vi "PolarizationSimulation_Final.vi"() -> ()   [LabVIEW 2019]
uses:
  <vilib>/Analysis/NI_AALBase.lvlib
  <vilib>/Utility/xml.llb/Write to XML File(string).vi
  <vilib>/Utility/xml.llb/Read From XML File(string).vi
  Integrated ANN/Sub-VIs/Adam_data.ctl
panel:
  out "Standard \nDeviation Noise":dbl step=0.0001
  out "NN Error":dbl
  out "NN Output":dbl
  out "Saturation\nPolarization":dbl=0.8 min=0.0 max=0.99 step=0.01
  out "Signal and Fit (P) 2":cluster{dbl[], "Best Polynomial Fit":dbl[]}[](graph)
  out "NN Graph":cluster{dbl[], dbl[]}(graph)
  in  "Regularization":T1
  in  "Batch Size":i16
  out "NN Loss":dbl(graph)
  in  "Loss Function":enum16{"MSE", "MAE"}(ring)
  in  "Parameters File Path":path
  out "NN Error":dbl
  in  "Training?":bool
  out "NN Output":dbl
  in  "Speed\nMultiplier":dbl=1.0
  in  "AFP On":bool
  in  "AFP Efficiency":dbl=0.9 min=0.0 max=1.0 step=0.01
  in  "AFP Control":cluster{i32, i32}(slide)={200, 230} scale=0.0..500.0
  out "lower R-value AFP":dbl
  out "upper R-value AFP":dbl
  in  "STOP":bool
  in  "Microwave Power":dbl=1.0
  in  "Lower Fit\nParameter":dbl=-3.6
  in  "Upper Fit\nParameter":dbl=3.6
  in  "Std Dev Noise":dbl step=0.0001
  out "lower R-value":dbl
  out "upper R-value":dbl
  in  "RF Control":cluster{i32, i32}(slide)={200, 230} scale=0.0..500.0
  out "p":dbl format="%_4g"
  out "r":dbl
  in  "Saturation\nPolarization":dbl=0.8 min=0.0 max=0.99 step=0.01
  out "Reimann \nsum of Q":dbl format="%_4g"
  out "Corrected Data (Q)":cluster{dbl[], dbl[]}(graph)
  in  "Select Target Type":u16(ring)=2 items=["Test Case", "Deuteron"]
  in  "Reset":bool
  out "Total Polarization (P)":cluster{dbl, dbl}(graph)
  in  "Spin Manipulation\nPower Factor":dbl=0.005
  in  "Decay Spin\nManipulation":bool
  out "Reimann\nsum of P":dbl format="%_4g"
  out "Corrected Data (P)":cluster{dbl[], dbl[]}[](graph)
  out "Signal and Fit (P)":cluster{dbl[], "Best Polynomial Fit":dbl[]}[](graph)
  in  "Positive\nPolarization":bool
  in  "Microwave on":bool
  # "Neural Network"
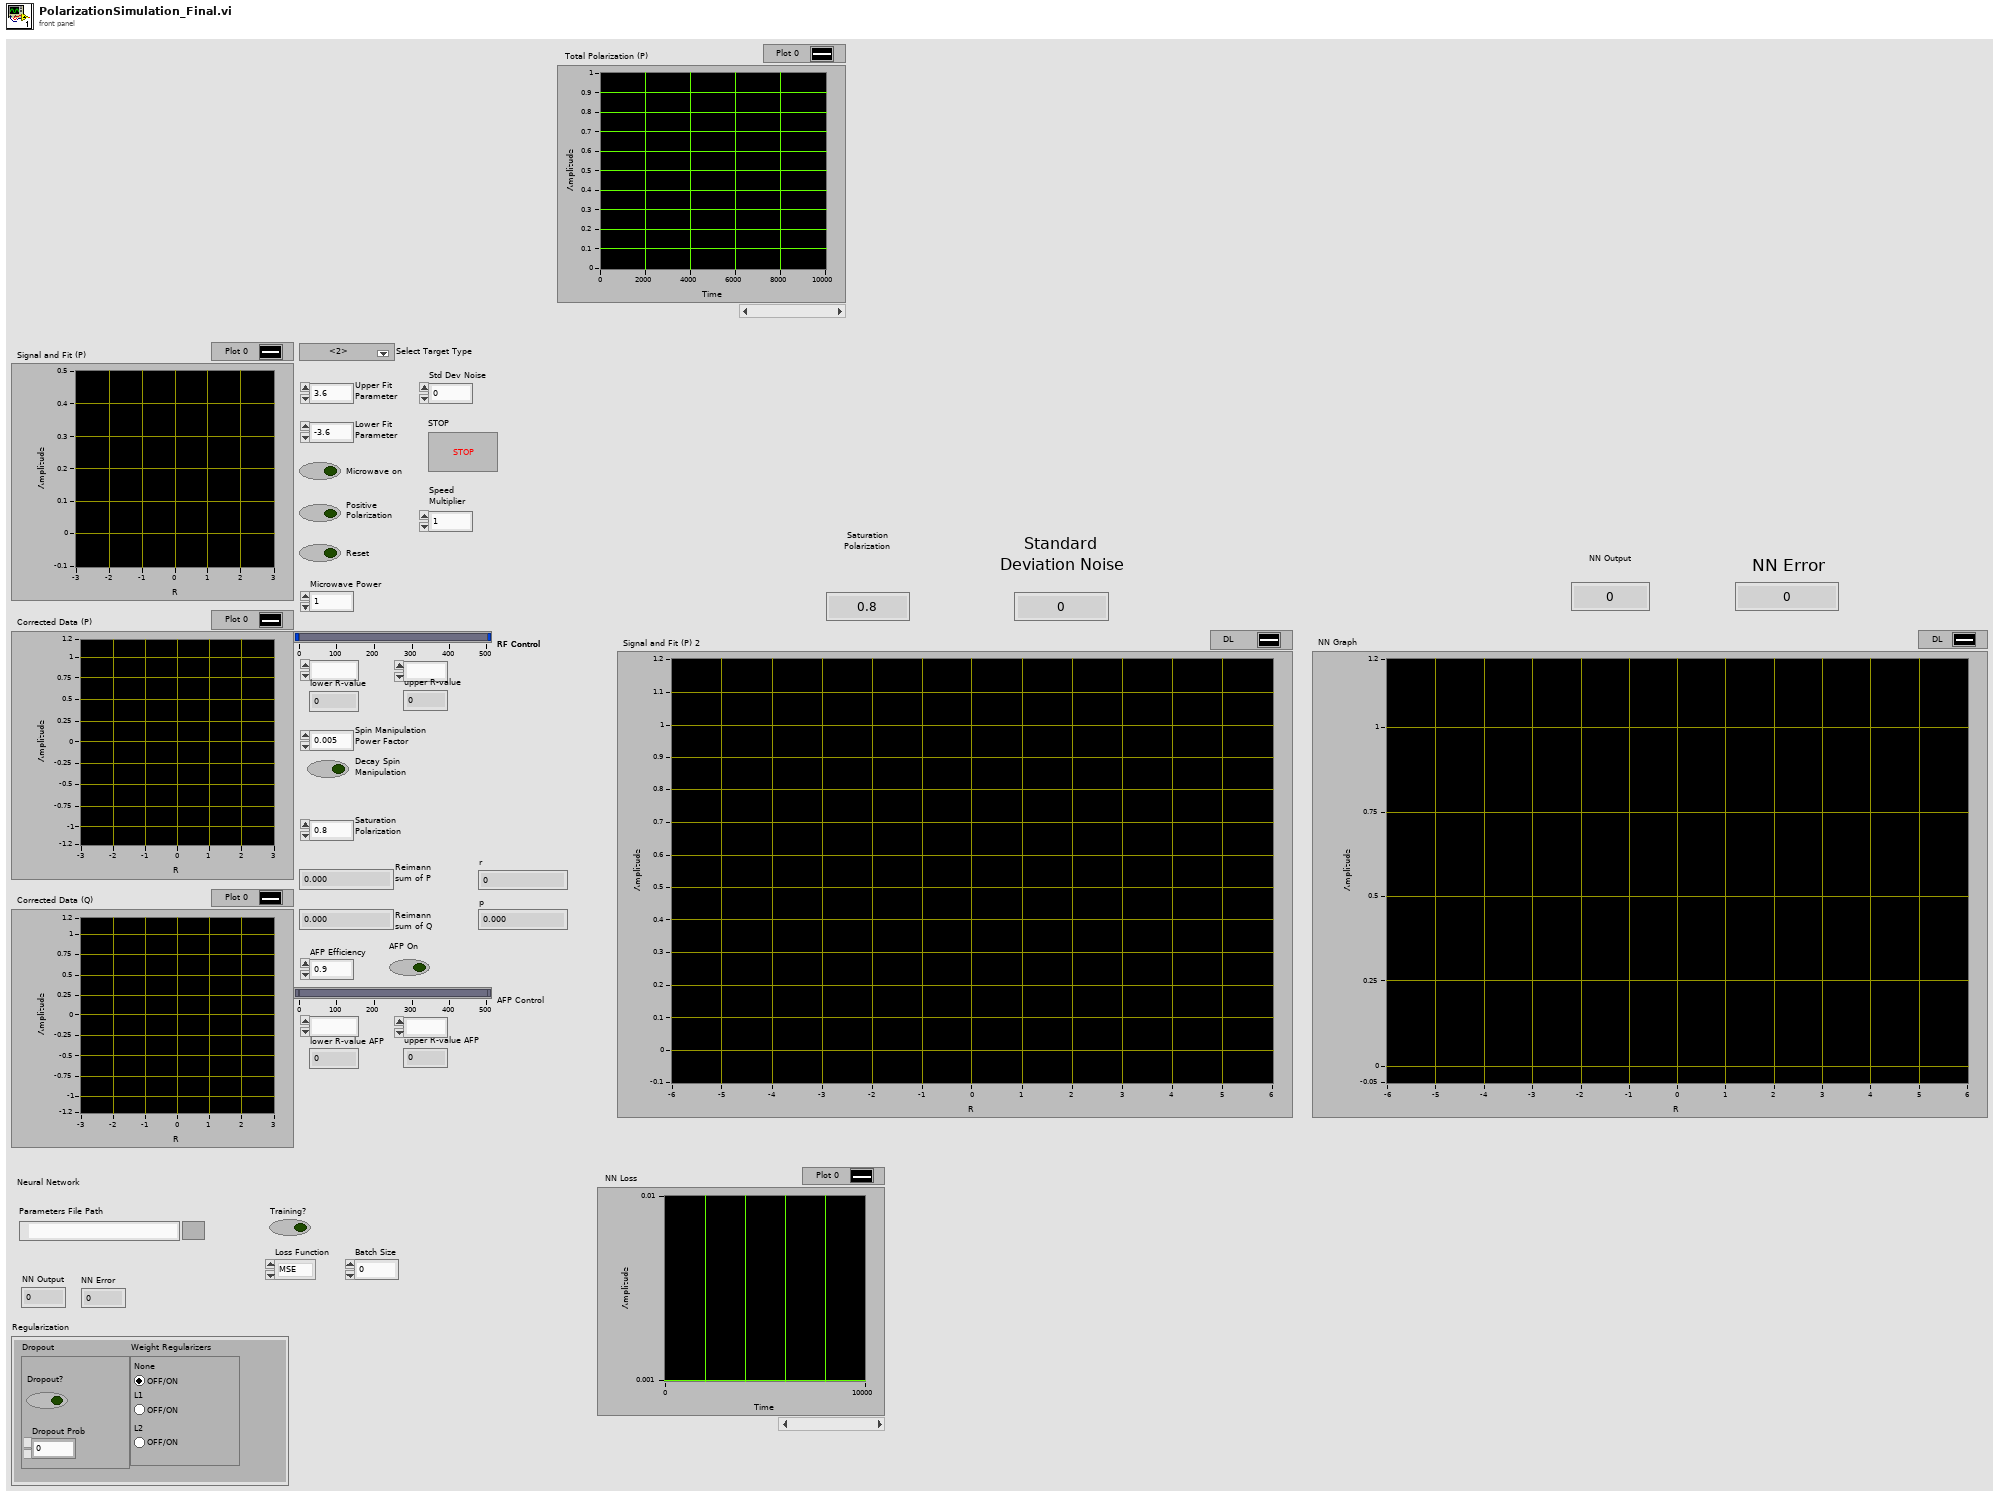
[diagram p1: front panel]
types:
  T1 = cluster{"Dropout":cluster{"Dropout?":bool, "Dropout Prob":dbl}, "Weight Regularizers":enum32{"None", "L1", "L2"}}
  T2 = typedef "Adam_data.ctl" = cluster{"Mw Moments":cluster{"3 ":dbl[], "2":dbl[][], "1":dbl[][]}, "Vw Moments":cluster{"3":dbl[], "2":dbl[][], "1":dbl[][]}, "Mb Moments":cluster{"3":dbl, "2":dbl[], "1":dbl[]}, "Vb Moments":cluster{"3":dbl, "2":dbl[], "1":dbl[]}}
  T3 = cluster{cluster{dbl[][], dbl[]}, cluster{dbl[][], dbl[]}, cluster{dbl[], dbl}}
  T4 = cluster{cluster{"Updated Weights":dbl[][], "Updated Biases":dbl[]}, cluster{"Updated Weights":dbl[][], "Updated Biases":dbl[]}, cluster{"Updated Weights":dbl[], "Updated Biases":dbl}}
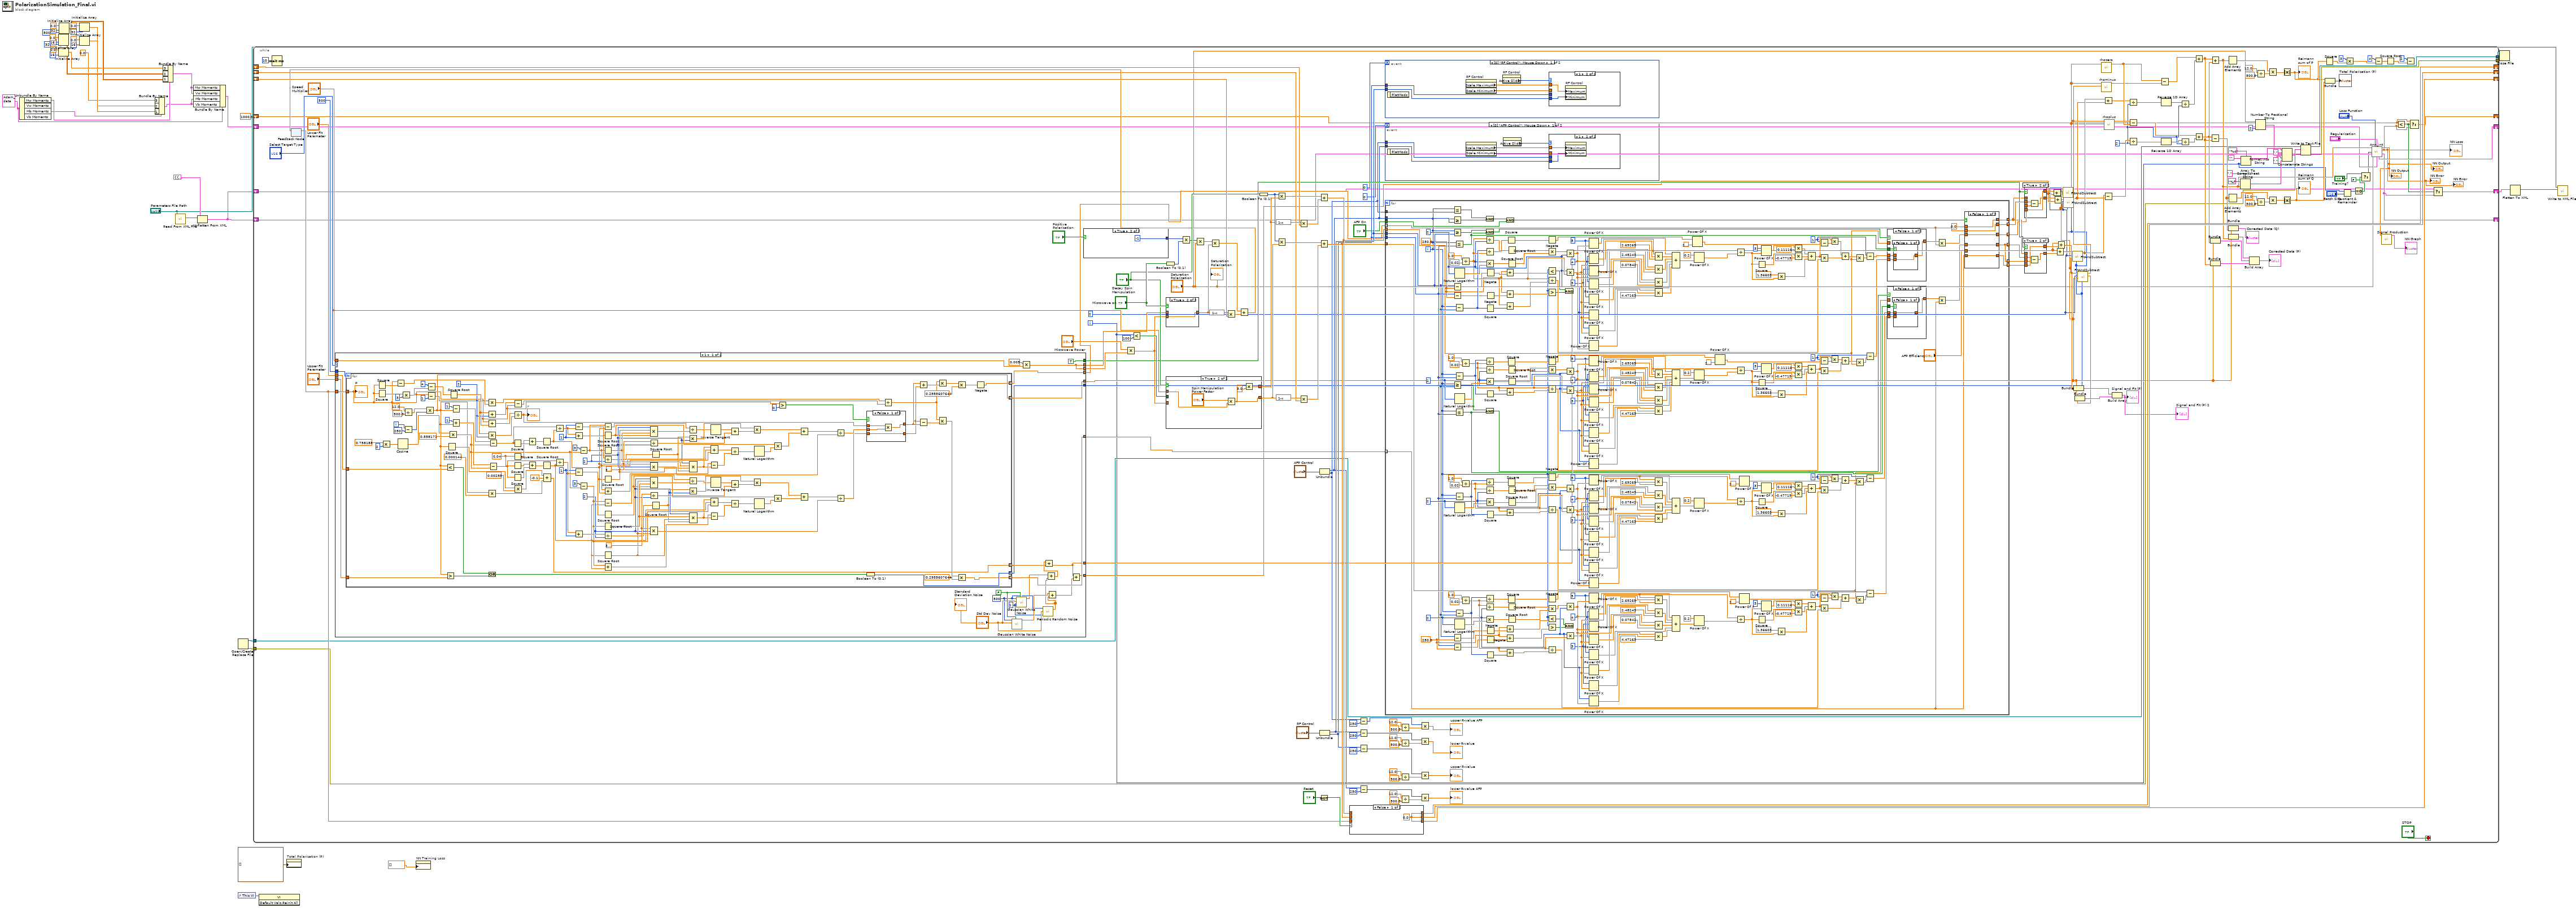
[diagram p0: block diagram]
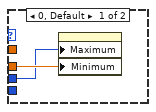
[diagram p2: hidden frame]
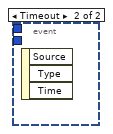
[diagram p3: hidden frame]
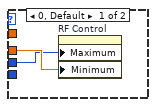
[diagram p4: hidden frame]
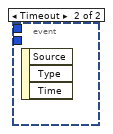
[diagram p5: hidden frame]
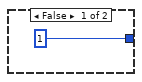
[diagram p6: hidden frame]
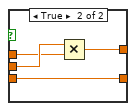
[diagram p7: hidden frame]
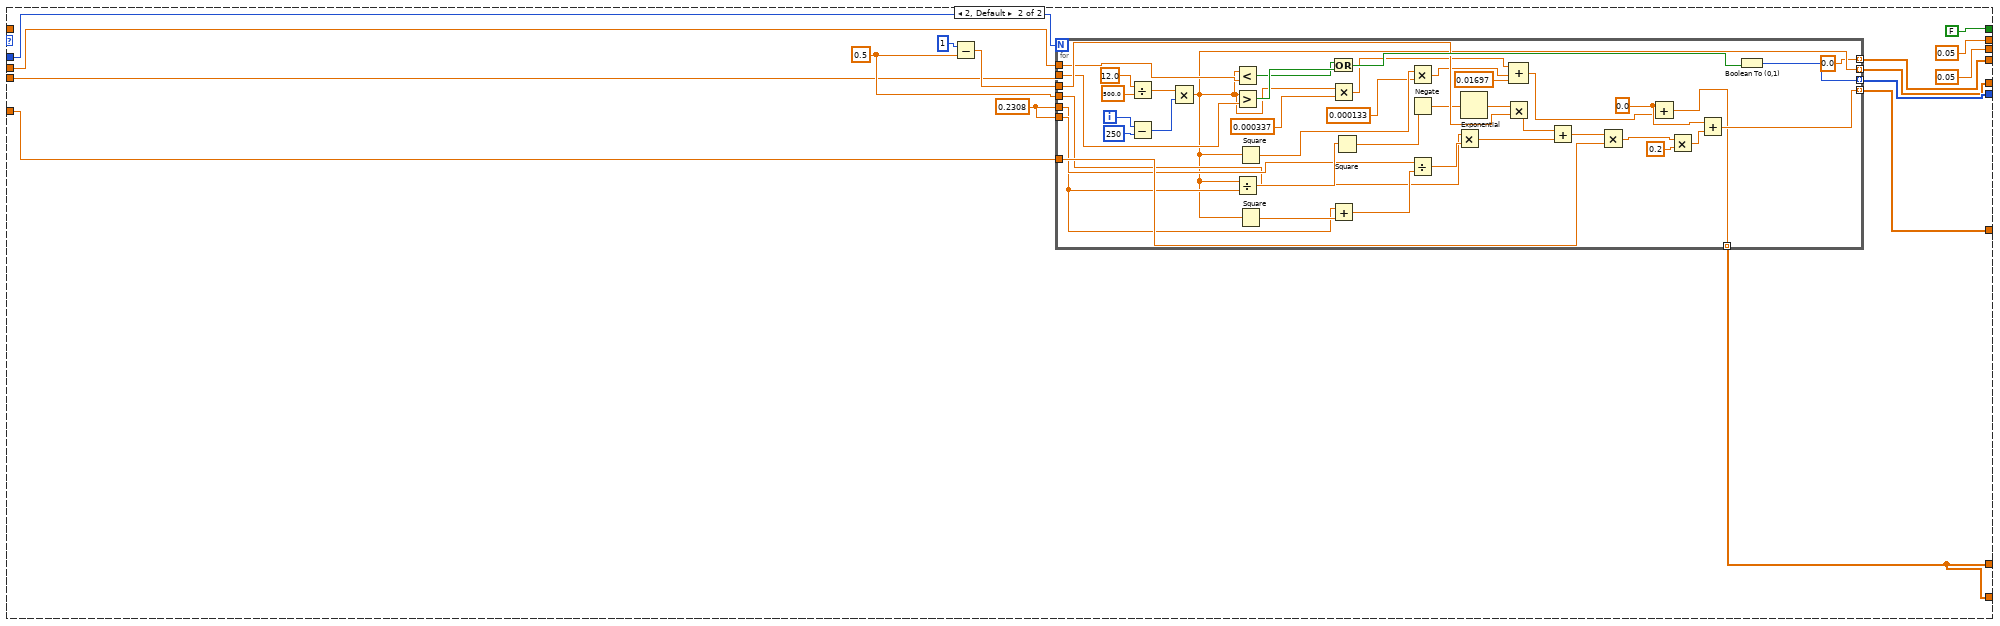
[diagram p8: hidden frame]
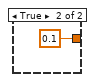
[diagram p10: hidden frame]
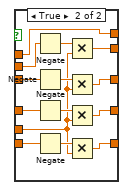
[diagram p15: hidden frame]
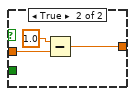
[diagram p17: hidden frame]
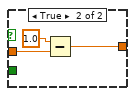
[diagram p19: hidden frame]
diagram:
  w7 = T2 {"Mw Moments"={"3 "=[], "2"=[], "1"=[]}, "Vw Moments"={"3"=[], "2"=[], "1"=[]}, "Mb Moments"={"3"=0.0, "2"=[], "1"=[]}, "Vb Moments"={"3"=0.0, "2"=[], "1"=[]}} ("Adam Data In")
  n1 = Unbundle By Name(w7) -> ("Mw Moments"=w9:cluster{"3 ":dbl[], "2":dbl[][], "1":dbl[][]}, "Mb Moments"=w8:cluster{"3":dbl, "2":dbl[], "1":dbl[]})  [unwired: 2 out]
  n2 = Initialize Array(0.0 ("element"), 16 ("dimension size"), 32 ("dimension size")) -> (w14:dbl[][])
  n3 = Initialize Array(0.0 ("element"), 16 ("dimension size")) -> (w13:dbl[])
  n4 = Initialize Array(0.0 ("element"), 32 ("dimension size"), 500 ("dimension size")) -> (w15:dbl[][])
  n5 = Initialize Array(0.0 ("element"), 16 ("dimension size")) -> (w11:dbl[])
  n6 = Initialize Array(0.0 ("element"), 32 ("dimension size")) -> (w12:dbl[])
  n7 = Bundle By Name(cluster=w8, "3"=0.0 ("element"), "2"=w11, "1"=w12) -> (w5:cluster{"3":dbl, "2":dbl[], "1":dbl[]})
  n8 = Bundle By Name(cluster=w9, "3"=w13, "2"=w14, "1"=w15) -> (w6:cluster{"3 ":dbl[], "2":dbl[][], "1":dbl[][]})
  n9 = call-poly <vilib>:"Read From XML File.vi"("XML File Path"="Parameters File Path") -> ("XML Elements"=w32:string)  [unwired: 8 in, 2 out]
  n10 = Bundle By Name(cluster=w7, "Mw Moments"=w6, "Vw Moments"=w6, "Mb Moments"=w5, "Vb Moments"=w5) -> (w4:T2)
  n11 = Unflatten From XML(xml string=w32, type=T3 {{[], []}, {[], []}, {[], 0.0}}) -> (value=w3:T3)  [unwired: 1 in, 1 out]
  n12 = Open/Create/Replace File() -> (refnum out=w36:refnum<file>, error out=w35:errorcluster)  [unwired: 6 in, 1 out]
  n13 = control-ref of="This VI"() -> (w38:refnum<vi>)
  n14 = while {
    shift-right: [w213] -> _
    shift-left: _ -> [w220]
    shift-right: [w212] -> _
    shift-left: _ -> [w195]
    shift-right: [w190] -> _
    shift-left: _ -> [w189]
    tunnel: w36 -> [w122]
    tunnel: w35 -> [w121]
    tunnel: [w120] -> w34
    tunnel: [w119] -> w33
    shift-right: [w46] -> _
    shift-left: w3 -> [w60]
    shift-right: [w58] -> _
    shift-left: w4 -> [w57]
    shift-right: [w49] -> _
    shift-left: 1000.0 ("Error") -> [w48]
    shift-right: [w45] -> w2
    shift-left: w3 -> [w44]
    i -> [w56]
    stop <- "STOP" stop-if-true
    w172 = 2
    w69 = 2
    n15 = Wait (ms)(milliseconds to wait=10) -> ()  [unwired: 1 out]
    n16 = feedback #1() -> (w199:dbl)  [unwired: 1 in]
    n17 = case shown="1" "Select Target Type" {
      tunnel: [w261 0.05 ("Growth Constant")] -> w204
      tunnel: [w261 0.05 ("Decay Constant")] -> w203
      tunnel: 500 -> [w267 w425]
      tunnel: w199 -> [w270 w424]
      tunnel: "Upper Fit\nParameter" -> [w268 w422]
      tunnel: "Lower Fit\nParameter" -> [w269 w423]
      tunnel: [w265 w420] -> w68
      tunnel: [w258 w419] -> w82
      tunnel: [w266 w421] -> w67
      tunnel: [TRUE FALSE] -> w183
      tunnel: [w259 w415] -> w81
      tunnel: "Speed\nMultiplier" -> [w260 _]
      tunnel: [w255 w414] -> w80
      tunnel: [w256 w414] -> w79
      frame 1 {
        w252 = 1
        w262 = FALSE
        w251 = 500
        n18 = for {
          N: w267 -> [_]
          tunnel: [w301] -> w265 mode=indexing
          tunnel: [w390] -> w266 mode=indexing
          tunnel: w268 -> [w389]
          tunnel: w269 -> [w388]
          tunnel: [w273] -> w258 mode=indexing
          tunnel: w270 -> [w274]
          tunnel: [w272] -> w259 mode=indexing
          tunnel: [w271] -> w257 mode=indexing
          i -> [w366]
          w288 = 2
          w327 = 1
          w331 = 3.141592653589793
          w325 = 2
          w310 = 0.04
          w363 = 1
          w368 = 3.141592653589793
          w361 = 2
          n19 = Square(x=w274) -> (x^2=w291:dbl)
          n20 = Square(x=w274) -> (x^2=w317:dbl)
          n21 = Multiply(x=0.758188, y=2) -> (x*y=w305:dbl)
          n22 = Subtract(x=w274, y=w291) -> (x-y=w290:dbl)
          n23 = Cosine(x=w305) -> (cos(x)=w308:dbl)
          n24 = Multiply(x=w317, y=3) -> (x*y=w316:dbl)
          n25 = Divide(x=12.0, y=500.0) -> (x/y=w404:dbl)
          n26 = Subtract(x=w366, y=250) -> (x-y=w403:i32)
          n27 = Multiply(x=w404, y=w403) -> (x*y=w301:dbl)
          n28 = Subtract(x=4, y=w316) -> (x-y=w314:dbl)
          n29 = Subtract(x=w274, y=1) -> (x-y=w312:dbl)
          n30 = Less?(x=w301, y=w388) -> (x < y?=w393:bool)
          n31 = Greater?(x=w301, y=w389) -> (0:w392:bool)
          n32 = Square(x=w301) -> (x^2=w303:dbl)
          n33 = Multiply(x=w308, y=0.558171) -> (x*y=w309:dbl)
          n34 = Square Root(x=w314) -> (sqrt(x)=w289:dbl)
          n35 = Subtract(x=1, y=w301) -> (x-y=w398:dbl)
          n36 = Add(x=1, y=w301) -> (x+y=w355:dbl)
          n37 = Multiply(x=w288, y=w290) -> (x*y=w286:dbl)
          n38 = Add(x=w289, y=w288) -> (x+y=w287:dbl)
          n39 = Add(x=w274, y=w289) -> (x+y=w313:dbl)
          n40 = Multiply(x=w312, y=w288) -> (x*y=w296:dbl)
          n41 = Multiply(x=w301, y=0.000144) -> (x*y=w298:dbl)
          n42 = Or(x=w393, y=w392) -> (x .or. y?=w391:bool)
          n43 = Subtract(x=w398, y=w309) -> (x-y=w394:dbl)
          n44 = Subtract(x=w355, y=w309) -> (x-y=w351:dbl)
          n45 = Square(x=w394) -> (x^2=w397:dbl)
          n46 = Square(x=w310) -> (x^2=w396:dbl)
          n47 = Square(x=w310) -> (x^2=w353:dbl)
          n48 = Square(x=w351) -> (x^2=w354:dbl)
          n49 = Subtract(x=w287, y=w274) -> (x-y=w285:dbl)
          n50 = Divide(x=w313, y=w296) -> (x/y=w292:dbl)
          "r" <- w292
          n51 = Multiply(x=w303, y=0.00295) -> (x*y=w302:dbl)
          n52 = Add(x=w396, y=w397) -> (x+y=w395:dbl)
          n53 = Add(x=w353, y=w354) -> (x+y=w352:dbl)
          n54 = Square Root(x=w395) -> (sqrt(x)=w358:dbl)
          n55 = Square Root(x=w352) -> (sqrt(x)=w322:dbl)
          n56 = Compound Arithmetic op=ADD(w302, -0.1, w298) -> (w271:dbl)
          n57 = Divide(x=w394, y=w358) -> (x/y=w364:dbl)
          n58 = Divide(x=w351, y=w322) -> (x/y=w328:dbl)
          n59 = Subtract(x=w363, y=w364) -> (x-y=w319:dbl)
          n60 = Add(x=w364, y=w363) -> (x+y=w362:dbl)
          n61 = Subtract(x=w327, y=w328) -> (x-y=w320:dbl)
          n62 = Add(x=w328, y=w327) -> (x+y=w326:dbl)
          n63 = Subtract(x=3, y=w309) -> (x-y=w374:dbl)
          n64 = Subtract(x=3, y=w309) -> (x-y=w337:dbl)
          n65 = Subtract(x=w374, y=w358) -> (x-y=w383:dbl)
          n66 = Square Root(x=w319) -> (sqrt(x)=w365:dbl)
          n67 = Square Root(x=w374) -> (sqrt(x)=w377:dbl)
          n68 = Divide(x=w362, y=w361) -> (x/y=w360:dbl)
          n69 = Square Root(x=w358) -> (sqrt(x)=w367:dbl)
          n70 = Add(x=w374, y=w358) -> (x+y=w373:dbl)
          n71 = Subtract(x=w337, y=w322) -> (x-y=w346:dbl)
          n72 = Square Root(x=w320) -> (sqrt(x)=w329:dbl)
          n73 = Square Root(x=w337) -> (sqrt(x)=w340:dbl)
          n74 = Divide(x=w326, y=w325) -> (x/y=w324:dbl)
          n75 = Square Root(x=w322) -> (sqrt(x)=w330:dbl)
          n76 = Add(x=w337, y=w322) -> (x+y=w336:dbl)
          n77 = Divide(x=w368, y=w361) -> (x/y=w385:dbl)
          n78 = Divide(x=w331, y=w325) -> (x/y=w348:dbl)
          n79 = Compound Arithmetic op=MULTIPLY(w361, w367, w377, w365) -> (w382:dbl)
          n80 = Compound Arithmetic op=MULTIPLY(w368, w361, w367) -> (w369:dbl)
          n81 = Compound Arithmetic op=MULTIPLY(w325, w330, w340, w329) -> (w345:dbl)
          n82 = Compound Arithmetic op=MULTIPLY(w331, w325, w330) -> (w332:dbl)
          n83 = Square Root(x=w360) -> (sqrt(x)=w359:dbl)
          n84 = Square Root(x=w324) -> (sqrt(x)=w323:dbl)
          n85 = Divide(x=w383, y=w382) -> (x/y=w381:dbl)
          n86 = Multiply(x=w359, y=w361) -> (x*y=w387:dbl)
          n87 = Divide(x=w346, y=w345) -> (x/y=w344:dbl)
          n88 = Multiply(x=w323, y=w325) -> (x*y=w350:dbl)
          n89 = Compound Arithmetic op=MULTIPLY(w361, w377, w367, w359) -> (w372:dbl)
          n90 = Compound Arithmetic op=MULTIPLY(w325, w340, w330, w323) -> (w335:dbl)
          n91 = Subtract(x=w373, y=w372) -> (x-y=w371:dbl)
          n92 = Subtract(x=w336, y=w335) -> (x-y=w334:dbl)
          n93 = Inverse Tangent(1:w381) -> (0:w386:dbl)
          n94 = Compound Arithmetic op=ADD(w372, w358, w374) -> (w376:dbl)
          n95 = Inverse Tangent(1:w344) -> (0:w349:dbl)
          n96 = Compound Arithmetic op=ADD(w335, w322, w337) -> (w339:dbl)
          n97 = Add(x=w386, y=w385) -> (x+y=w384:dbl)
          n98 = Divide(x=w376, y=w371) -> (x/y=w375:dbl)
          n99 = Add(x=w349, y=w348) -> (x+y=w347:dbl)
          n100 = Divide(x=w339, y=w334) -> (x/y=w338:dbl)
          n101 = Multiply(x=w387, y=w384) -> (x*y=w380:dbl)
          n102 = Multiply(x=w350, y=w347) -> (x*y=w343:dbl)
          n103 = Natural Logarithm(1:w375) -> (0:w378:dbl)
          n104 = Natural Logarithm(1:w338) -> (0:w341:dbl)
          n105 = Multiply(x=w365, y=w378) -> (x*y=w379:dbl)
          n106 = Multiply(x=w329, y=w341) -> (x*y=w342:dbl)
          n107 = Greater?(x=w274, y=0) -> (0:w276:bool)
          n108 = Add(x=w380, y=w379) -> (x+y=w370:dbl)
          n109 = Add(x=w343, y=w342) -> (x+y=w333:dbl)
          n110 = Divide(x=w370, y=w369) -> (x/y=w311:dbl)
          n111 = Divide(x=w333, y=w332) -> (x/y=w278:dbl)
          n112 = Boolean To (0,1)(Boolean=w391) -> (0, 1=w390:i16)
          n113 = case shown="False" w276 {
            tunnel: w311 -> [w408 w413]
            tunnel: [w406 w412] -> w294
            tunnel: w292 -> [w409 w411]
            tunnel: w278 -> [w407 w410]
            tunnel: [w407 w410] -> w277
            frame False {
              n114 = Multiply(x=w409, y=w408) -> (x*y=w406:dbl)
            }
            frame True {
              n115 = Multiply(x=w413, y=w411) -> (x*y=w412:dbl)
            }
          }
          n116 = Divide(x=w286, y=w285) -> (x/y=w284:dbl)
          n117 = Add(x=w294, y=w277) -> (x+y=w295:dbl)
          n118 = Subtract(x=w277, y=w294) -> (x-y=w321:dbl)
          n119 = Multiply(x=w284, y=w295) -> (x*y=w283:dbl)
          n120 = Multiply(x=w284, y=w321) -> (x*y=w282:dbl)
          n121 = Multiply(x=w283, y=0.2955607644) -> (x*y=w281:dbl)
          n122 = Multiply(x=w282, y=0.2955607644) -> (x*y=w273:dbl)
          n123 = Negate(x=w281) -> (-x=w272:dbl)
          "p" <- w274
        }
        n124 = call <vilib>:"Gaussian White Noise.vi"("initialize?"=w262, "standard deviation"="Std Dev Noise", "samples"=w251) -> ("Gaussian noise pattern"=w253:dbl[])  [unwired: 7 in, 1 out]
        n125 = call <vilib>:"Gaussian White Noise.vi"("initialize?"=w262, "seed"=w252, "standard deviation"="Std Dev Noise", "samples"=w251) -> ("Gaussian noise pattern"=w248:dbl[])  [unwired: 6 in, 1 out]
        n126 = Multiply(x=0.005, y=w260) -> (x*y=w261:dbl)
        n127 = call <vilib>:"Periodic Random Noise.vi"("seed"=w252, "spectral amplitude"="Std Dev Noise", "samples"=w251) -> ("periodic random noise"=w249:dbl[])  [unwired: 1 out]
        n128 = Add(x=w248, y=w249) -> (x+y=w247:dbl[])
        n129 = Add(x=w247, y=w257) -> (x+y=w255:dbl[])
        n130 = Add(x=w253, y=w249) -> (x+y=w250:dbl[])
        n131 = Add(x=w255, y=w250) -> (x+y=w256:dbl[])
        "Standard \nDeviation Noise" <- "Std Dev Noise"
      }
      frame 2, Default {
        w426 = 0.2308
        w427 = 0.5
        n132 = Subtract(x=1, y=w427) -> (x-y=w429:dbl)
        n133 = for {
          N: w425 -> [_]
          tunnel: w424 -> [w469]
          tunnel: [w435] -> w420 mode=indexing
          tunnel: [w453] -> w419 mode=indexing
          tunnel: [w467] -> w421 mode=indexing
          tunnel: w429 -> [w463]
          tunnel: w426 -> [w461]
          tunnel: w426 -> [w442]
          tunnel: w427 -> [w455]
          tunnel: w422 -> [w450]
          tunnel: w423 -> [w449]
          tunnel: [0.0] -> w415 mode=indexing
          tunnel: [w430] -> w414 mode=indexing
          i -> [w443]
          w454 = 0.0
          n134 = Divide(x=12.0, y=500.0) -> (x/y=w444:dbl)
          n135 = Subtract(x=w443, y=250) -> (x-y=w448:i32)
          n136 = Multiply(x=w444, y=w448) -> (x*y=w435:dbl)
          n137 = Less?(x=w435, y=w449) -> (x < y?=w464:bool)
          n138 = Greater?(x=w435, y=w450) -> (0:w465:bool)
          n139 = Divide(x=w435, y=w442) -> (x/y=w470:dbl)
          n140 = Square(x=w435) -> (x^2=w438:dbl)
          n141 = Square(x=w435) -> (x^2=w460:dbl)
          n142 = Or(x=w464, y=w465) -> (x .or. y?=w466:bool)
          n143 = Multiply(x=w435, y=0.000337) -> (x*y=w437:dbl)
          n144 = Add(x=w442, y=w460) -> (x+y=w462:dbl)
          n145 = Square(x=w470) -> (x^2=w471:dbl)
          n146 = Multiply(x=w438, y=0.000133) -> (x*y=w436:dbl)
          n147 = Negate(x=w471) -> (-x=w452:dbl)
          n148 = Divide(x=w461, y=w462) -> (x/y=w457:dbl)
          n149 = Multiply(x=w455, y=w457) -> (x*y=w456:dbl)
          n150 = Exponential(1:w452) -> (0:w451:dbl)
          n151 = Multiply(x=w451, y=w463) -> (x*y=w459:dbl)
          n152 = Compound Arithmetic op=ADD(w437, w436, 0.01697) -> (w439:dbl)
          n153 = Add(x=w459, y=w456) -> (x+y=w458:dbl)
          n154 = Multiply(x=w458, y=w469) -> (x*y=w468:dbl)
          n155 = Add(x=w454, y=w439) -> (x+y=w430:dbl)
          n156 = Multiply(x=w468, y=0.2) -> (x*y=w441:dbl)
          n157 = Add(x=w454, y=w441) -> (x+y=w453:dbl)
          n158 = Boolean To (0,1)(Boolean=w466) -> (0, 1=w467:i16)
        }
      }
    }
    n159 = case shown="True" "Positive\nPolarization" {
      tunnel: [1 -1] -> w157
      frame False {
      }
      frame True {
      }
    }
    n160 = Multiply(x="Microwave Power", y=w204) -> (x*y=w125:dbl)
    n161 = Less?(x=w56, y=100) -> (x < y?=w215:bool)
    n162 = Boolean To (0,1)(Boolean="Microwave on") -> (0, 1=w222:i16)
    n163 = case shown="True" "Microwave on" {
      tunnel: [w482 w483] -> w207
      tunnel: w125 -> [_ w483]
      tunnel: w203 -> [w482 _]
      frame False {
      }
      frame True {
      }
    }
    n164 = case shown="True" "Decay Spin\nManipulation" {
      tunnel: [w472 w478] -> w216
      tunnel: w125 -> [w474 _]
      tunnel: w215 -> [w473 _]
      tunnel: [w472 w479] -> w197
      tunnel: "Speed\nMultiplier" -> [_ w477]
      frame False {
        n165 = case shown="False" w473 {
          tunnel: [w475 0.1] -> w472
          tunnel: w474 -> [w475 _]
          frame False {
          }
          frame True {
          }
        }
      }
      frame True {
        n166 = Multiply(x="Spin Manipulation\nPower Factor", y=w477) -> (x*y=w478:dbl)
        n167 = Multiply(x=w478, y=3.0) -> (x*y=w479:dbl)
      }
    }
    n168 = Multiply(x=w157, y=w222) -> (x*y=w158:i32)
    n169 = Multiply(x=w158, y="Saturation\nPolarization") -> (x*y=w165:dbl)
    n170 = expression code="1-x"(w207) -> (w223:dbl)
    n171 = Multiply(x=w165, y=w207) -> (x*y=w224:dbl)
    n172 = Multiply(x=w223, y=w220) -> (x*y=w225:dbl)
    n173 = Add(x=w224, y=w225) -> (x+y=w202:dbl)
    n174 = feedback-in #1(w202) -> ()
    n175 = Boolean To (0,1)(Boolean="Decay Spin\nManipulation") -> (0, 1=w198:i16)
    n176 = expression code="1-x"(w197) -> (w196:dbl)
    n177 = expression code="1-x"(w216) -> (w217:dbl)
    n178 = Multiply(x=w198, y=w197) -> (x*y=w193:dbl)
    n179 = Multiply(x=w198, y=w216) -> (x*y=w218:dbl)
    n180 = Multiply(x=w196, y=w189) -> (x*y=w194:dbl)
    n181 = Multiply(x=w217, y=w195) -> (x*y=w219:dbl)
    n182 = Add(x=w193, y=w194) -> (x+y=w191:dbl)
    n183 = Add(x=w218, y=w219) -> (x+y=w211:dbl)
    n184 = Not(x="Reset") -> (.not. x?=w210:bool)
    n185 = Unbundle("AFP Control") -> (w89:i32, w88:i32)
    n186 = Unbundle("RF Control") -> (w128:i32, w127:i32)
    n187 = case shown="False" w210 {
      tunnel: [w496 w499] -> w213
      tunnel: w199 -> [_ w499]
      tunnel: [w496 w498] -> w212
      tunnel: w211 -> [_ w498]
      tunnel: w191 -> [_ w497]
      tunnel: [w496 w497] -> w190
      frame False {
        w496 = 0.0
      }
      frame True {
      }
    }
    n188 = Subtract(x=w88, y=250) -> (x-y=w95:i32)
    n189 = Subtract(x=w128, y=250) -> (x-y=w134:i32)
    n190 = Subtract(x=w127, y=250) -> (x-y=w137:i32)
    n191 = Subtract(x=w89, y=250) -> (x-y=w92:i32)
    n192 = event shown="[0] \"RF Control\": Mouse Down" {
      selector: _ -> [_ _]
      dyn-events: _ -> [_ _]
      timeout: 0 -> [_ _]
      tunnel: w128 -> [w237 _]
      tunnel: w127 -> [w236 _]
      event "RF Control": Mouse Down {
        n193 = event-data() -> ()  [unwired: 1 in, 1 out]
        n194 = property on="RF Control" class="Slide (strict)"() -> ("Scale.Maximum"=w238:dbl, "Scale.Minimum"=w239:dbl)  [unwired: 2 in, 2 out]
        n195 = property on="RF Control" class="Slide (strict)"() -> ("Active Slider"=w240:i32)  [unwired: 2 in, 2 out]
        n196 = case shown="1" w240 {
          tunnel: w239 -> [w242 _]
          tunnel: w236 -> [w241 _]
          tunnel: w238 -> [_ w244]
          tunnel: w237 -> [_ w243]
          frame 0, Default {
            n197 = property on="RF Control" class="Slide (strict)"("Maximum"=w241, "Minimum"=w242) -> ()  [unwired: 2 in, 2 out]
          }
          frame 1 {
            n198 = property on="RF Control" class="Slide (strict)"("Maximum"=w244, "Minimum"=w243) -> ()  [unwired: 2 in, 2 out]
          }
        }
      }
      event Timeout {
        n199 = event-data() -> ()  [unwired: 1 in, 3 out]
      }
    }
    n200 = event shown="[0] \"AFP Control\": Mouse Down" {
      selector: _ -> [_ _]
      dyn-events: _ -> [_ _]
      timeout: 0 -> [_ _]
      tunnel: w89 -> [w228 _]
      tunnel: w88 -> [w227 _]
      event "AFP Control": Mouse Down {
        n201 = event-data() -> ()  [unwired: 1 in, 1 out]
        n202 = property on="AFP Control" class="Slide (strict)"() -> ("Scale.Maximum"=w229:dbl, "Scale.Minimum"=w230:dbl)  [unwired: 2 in, 2 out]
        n203 = property on="AFP Control" class="Slide (strict)"() -> ("Active Slider"=w231:i32)  [unwired: 2 in, 2 out]
        n204 = case shown="1" w231 {
          tunnel: w230 -> [w233 _]
          tunnel: w227 -> [w232 _]
          tunnel: w229 -> [_ w235]
          tunnel: w228 -> [_ w234]
          frame 0, Default {
            n205 = property on="AFP Control" class="Slide (strict)"("Maximum"=w232, "Minimum"=w233) -> ()  [unwired: 2 in, 2 out]
          }
          frame 1 {
            n206 = property on="AFP Control" class="Slide (strict)"("Maximum"=w235, "Minimum"=w234) -> ()  [unwired: 2 in, 2 out]
          }
        }
      }
      event Timeout {
        n207 = event-data() -> ()  [unwired: 1 in, 3 out]
      }
    }
    n208 = for {
      tunnel: w82 -> [w512] mode=indexing
      tunnel: w211 -> [w664]
      tunnel: w127 -> [w522]
      tunnel: w128 -> [w521]
      tunnel: [w508] -> w201 mode=indexing
      tunnel: [w509] -> w192 mode=indexing
      tunnel: [w509] -> w200 mode=indexing
      tunnel: w81 -> [w501] mode=indexing
      tunnel: w191 -> [w520]
      tunnel: [w500] -> w187 mode=indexing
      tunnel: [w507] -> w177 mode=indexing
      tunnel: w89 -> [w516]
      tunnel: w88 -> [w515]
      tunnel: "AFP On" -> [w504]
      tunnel: [w503] -> w86 mode=indexing
      i -> [w514]
      w524 = 250.0
      w563 = 5
      w561 = 4
      w560 = 3
      w541 = 1
      w542 = 2
      w624 = 5
      w622 = 4
      w621 = 3
      w601 = 1
      w602 = 2
      w658 = 250.0
      w699 = 5
      w697 = 4
      w696 = 3
      w677 = 1
      w678 = 2
      w760 = 5
      w758 = 4
      w757 = 3
      w737 = 1
      w738 = 2
      n209 = Less Or Equal?(x=w514, y=w515) -> (x <= y?=w517:bool)
      n210 = Greater Or Equal?(x=w514, y=w516) -> (x >= y?=w518:bool)
      n211 = Greater Or Equal?(x=w514, y=w521) -> (x >= y?=w597:bool)
      n212 = Subtract(x=w521, y=w524) -> (x-y=w528:dbl)
      n213 = Subtract(x=w522, y=w524) -> (x-y=w529:dbl)
      n214 = Greater Or Equal?(x=w514, y=w521) -> (x >= y?=w733:bool)
      n215 = Subtract(x=w521, y=w658) -> (x-y=w662:dbl)
      n216 = Subtract(x=w522, y=w658) -> (x-y=w663:dbl)
      n217 = Less Or Equal?(x=w514, y=w522) -> (x <= y?=w534:bool)
      n218 = Natural Logarithm(1:w602) -> (0:w637:dbl)
      n219 = Subtract(x=w514, y=w521) -> (x-y=w610:i32)
      n220 = Subtract(x=w514, y=w522) -> (x-y=w549:i32)
      n221 = Natural Logarithm(1:w542) -> (0:w576:dbl)
      n222 = Less Or Equal?(x=w514, y=w522) -> (x <= y?=w669:bool)
      n223 = Subtract(x=w514, y=w522) -> (x-y=w685:i32)
      n224 = Natural Logarithm(1:w678) -> (0:w712:dbl)
      n225 = Subtract(x=w514, y=w521) -> (x-y=w746:i32)
      n226 = Natural Logarithm(1:w738) -> (0:w773:dbl)
      n227 = Divide(x=1.0, y=0.02) -> (x/y=w606:dbl)
      n228 = Divide(x=1.0, y=0.02) -> (x/y=w546:dbl)
      n229 = Divide(x=1.0, y=0.02) -> (x/y=w682:dbl)
      n230 = Divide(x=1.0, y=0.02) -> (x/y=w742:dbl)
      n231 = And(x=w517, y=w518) -> (x .and. y?=w506:bool)
      n232 = And(x=w597, y=w534) -> (x .and. y?=w535:bool)
      n233 = Divide(x=w606, y=w602) -> (x/y=w635:dbl)
      n234 = Divide(x=w610, y=w606) -> (x/y=w614:dbl)
      n235 = Multiply(x=w602, y=w637) -> (x*y=w638:dbl)
      n236 = Divide(x=w549, y=w546) -> (x/y=w553:dbl)
      n237 = Divide(x=w546, y=w542) -> (x/y=w574:dbl)
      n238 = Multiply(x=w542, y=w576) -> (x*y=w577:dbl)
      n239 = And(x=w733, y=w669) -> (x .and. y?=w671:bool)
      n240 = Divide(x=w685, y=w682) -> (x/y=w689:dbl)
      n241 = Divide(x=w682, y=w678) -> (x/y=w710:dbl)
      n242 = Multiply(x=w678, y=w712) -> (x*y=w713:dbl)
      n243 = Divide(x=w746, y=w742) -> (x/y=w750:dbl)
      n244 = Divide(x=w742, y=w738) -> (x/y=w771:dbl)
      n245 = Multiply(x=w738, y=w773) -> (x*y=w774:dbl)
      n246 = Square(x=w610) -> (x^2=w611:i32)
      n247 = Square(x=w549) -> (x^2=w550:i32)
      n248 = Square(x=w685) -> (x^2=w686:i32)
      n249 = Square(x=w746) -> (x^2=w747:i32)
      n250 = Negate(x=w528) -> (-x=w527:dbl)
      n251 = Negate(x=w529) -> (-x=w525:dbl)
      n252 = Negate(x=w662) -> (-x=w661:dbl)
      n253 = Negate(x=w663) -> (-x=w659:dbl)
      n254 = Add(x=w524, y=w527) -> (x+y=w526:dbl)
      n255 = Add(x=w524, y=w525) -> (x+y=w523:dbl)
      n256 = Add(x=w606, y=w611) -> (x+y=w612:dbl)
      n257 = Add(x=w546, y=w550) -> (x+y=w551:dbl)
      n258 = Add(x=w682, y=w686) -> (x+y=w687:dbl)
      n259 = Add(x=w658, y=w661) -> (x+y=w660:dbl)
      n260 = Add(x=w658, y=w659) -> (x+y=w657:dbl)
      n261 = Add(x=w742, y=w747) -> (x+y=w748:dbl)
      n262 = And(x=w506, y=w504) -> (x .and. y?=w505:bool)
      n263 = Square(x=w614) -> (x^2=w616:dbl)
      n264 = Square(x=w553) -> (x^2=w555:dbl)
      n265 = Square(x=w689) -> (x^2=w691:dbl)
      n266 = Square(x=w750) -> (x^2=w752:dbl)
      n267 = Square Root(x=w635) -> (sqrt(x)=w636:dbl)
      n268 = Square Root(x=w638) -> (sqrt(x)=w639:dbl)
      n269 = Square Root(x=w574) -> (sqrt(x)=w575:dbl)
      n270 = Square Root(x=w577) -> (sqrt(x)=w578:dbl)
      n271 = Square Root(x=w710) -> (sqrt(x)=w711:dbl)
      n272 = Square Root(x=w713) -> (sqrt(x)=w714:dbl)
      n273 = Square Root(x=w771) -> (sqrt(x)=w772:dbl)
      n274 = Square Root(x=w774) -> (sqrt(x)=w775:dbl)
      n275 = Negate(x=w616) -> (-x=w615:dbl)
      n276 = Multiply(x=w636, y=w639) -> (x*y=w630:dbl)
      n277 = Less?(x=w514, y=w526) -> (x < y?=w531:bool)
      n278 = Divide(x=w606, y=w612) -> (x/y=w609:dbl)
      n279 = Greater?(x=w514, y=w523) -> (0:w530:bool)
      n280 = Negate(x=w555) -> (-x=w554:dbl)
      n281 = Multiply(x=w575, y=w578) -> (x*y=w569:dbl)
      n282 = Divide(x=w546, y=w551) -> (x/y=w536:dbl)
      n283 = Negate(x=w691) -> (-x=w690:dbl)
      n284 = Multiply(x=w711, y=w714) -> (x*y=w705:dbl)
      n285 = Divide(x=w682, y=w687) -> (x/y=w672:dbl)
      n286 = Negate(x=w752) -> (-x=w751:dbl)
      n287 = Multiply(x=w772, y=w775) -> (x*y=w766:dbl)
      n288 = Less?(x=w514, y=w660) -> (x < y?=w666:bool)
      n289 = Greater?(x=w514, y=w657) -> (0:w665:bool)
      n290 = Divide(x=w742, y=w748) -> (x/y=w745:dbl)
      n291 = And(x=w531, y=w530) -> ()  [unwired: 1 out]
      n292 = And(x=w666, y=w665) -> ()  [unwired: 1 out]
      n293 = Multiply(x=w630, y=w602) -> (x*y=w654:dbl)
      n294 = Multiply(x=w602, y=w606) -> (x*y=w648:dbl)
      n295 = Multiply(x=w569, y=w542) -> (x*y=w593:dbl)
      n296 = Multiply(x=w542, y=w546) -> (x*y=w587:dbl)
      n297 = Multiply(x=w705, y=w678) -> (x*y=w729:dbl)
      n298 = Multiply(x=w678, y=w682) -> (x*y=w723:dbl)
      n299 = Multiply(x=w766, y=w738) -> (x*y=w790:dbl)
      n300 = Multiply(x=w738, y=w742) -> (x*y=w784:dbl)
      n301 = Power Of X(1:w654, 2:w624) -> (0:w641:dbl)
      n302 = Power Of X(1:w654, 2:w622) -> (0:w647:dbl)
      n303 = Power Of X(1:w654, 2:w621) -> (0:w649:dbl)
      n304 = Power Of X(1:w648, 2:w622) -> (0:w653:dbl)
      n305 = Power Of X(1:w648, 2:w624) -> (0:w642:dbl)
      n306 = Power Of X(1:w648, 2:w602) -> (0:w650:dbl)
      n307 = Power Of X(1:w648, 2:w621) -> (0:w651:dbl)
      n308 = Power Of X(1:w654, 2:w602) -> (0:w652:dbl)
      n309 = Power Of X(1:w593, 2:w563) -> (0:w580:dbl)
      n310 = Power Of X(1:w593, 2:w561) -> (0:w586:dbl)
      n311 = Power Of X(1:w593, 2:w560) -> (0:w588:dbl)
      n312 = Power Of X(1:w587, 2:w561) -> (0:w592:dbl)
      n313 = Power Of X(1:w587, 2:w563) -> (0:w581:dbl)
      n314 = Power Of X(1:w587, 2:w542) -> (0:w589:dbl)
      n315 = Power Of X(1:w587, 2:w560) -> (0:w590:dbl)
      n316 = Power Of X(1:w593, 2:w542) -> (0:w591:dbl)
      n317 = Power Of X(1:w729, 2:w699) -> (0:w716:dbl)
      n318 = Power Of X(1:w729, 2:w697) -> (0:w722:dbl)
      n319 = Power Of X(1:w729, 2:w696) -> (0:w724:dbl)
      n320 = Power Of X(1:w723, 2:w697) -> (0:w728:dbl)
      n321 = Power Of X(1:w723, 2:w699) -> (0:w717:dbl)
      n322 = Power Of X(1:w723, 2:w678) -> (0:w725:dbl)
      n323 = Power Of X(1:w723, 2:w696) -> (0:w726:dbl)
      n324 = Power Of X(1:w729, 2:w678) -> (0:w727:dbl)
      n325 = Power Of X(1:w790, 2:w760) -> (0:w777:dbl)
      n326 = Power Of X(1:w790, 2:w758) -> (0:w783:dbl)
      n327 = Power Of X(1:w790, 2:w757) -> (0:w785:dbl)
      n328 = Power Of X(1:w784, 2:w758) -> (0:w789:dbl)
      n329 = Power Of X(1:w784, 2:w760) -> (0:w778:dbl)
      n330 = Power Of X(1:w784, 2:w738) -> (0:w786:dbl)
      n331 = Power Of X(1:w784, 2:w757) -> (0:w787:dbl)
      n332 = Power Of X(1:w790, 2:w738) -> (0:w788:dbl)
      n333 = Compound Arithmetic op=MULTIPLY(w648, w647, 2.69269) -> (w643:dbl)
      n334 = Compound Arithmetic op=MULTIPLY(w649, w650, 2.48243) -> (w645:dbl)
      n335 = Compound Arithmetic op=MULTIPLY(w654, w653, 0.07842) -> (w644:dbl)
      n336 = Compound Arithmetic op=MULTIPLY(w651, w652, 4.47163) -> (w646:dbl)
      n337 = Compound Arithmetic op=MULTIPLY(w587, w586, 2.69269) -> (w582:dbl)
      n338 = Compound Arithmetic op=MULTIPLY(w588, w589, 2.48243) -> (w584:dbl)
      n339 = Compound Arithmetic op=MULTIPLY(w593, w592, 0.07842) -> (w583:dbl)
      n340 = Compound Arithmetic op=MULTIPLY(w590, w591, 4.47163) -> (w585:dbl)
      n341 = Compound Arithmetic op=MULTIPLY(w723, w722, 2.69269) -> (w718:dbl)
      n342 = Compound Arithmetic op=MULTIPLY(w724, w725, 2.48243) -> (w720:dbl)
      n343 = Compound Arithmetic op=MULTIPLY(w729, w728, 0.07842) -> (w719:dbl)
      n344 = Compound Arithmetic op=MULTIPLY(w726, w727, 4.47163) -> (w721:dbl)
      n345 = Compound Arithmetic op=MULTIPLY(w784, w783, 2.69269) -> (w779:dbl)
      n346 = Compound Arithmetic op=MULTIPLY(w785, w786, 2.48243) -> (w781:dbl)
      n347 = Compound Arithmetic op=MULTIPLY(w790, w789, 0.07842) -> (w780:dbl)
      n348 = Compound Arithmetic op=MULTIPLY(w787, w788, 4.47163) -> (w782:dbl)
      n349 = Compound Arithmetic op=unknown(w641, w643, w645, w644, w642, w646) -> (w603:dbl)
      n350 = Compound Arithmetic op=unknown(w580, w582, w584, w583, w581, w585) -> (w543:dbl)
      n351 = Compound Arithmetic op=unknown(w716, w718, w720, w719, w717, w721) -> (w679:dbl)
      n352 = Compound Arithmetic op=unknown(w777, w779, w781, w780, w778, w782) -> (w739:dbl)
      n353 = Power Of X(1:2.718281828459045, 2:w615) -> (0:w613:dbl)
      n354 = Power Of X(1:w603, 2:0.2) -> (0:w656:dbl)
      n355 = Power Of X(1:w543, 2:0.2) -> (0:w595:dbl)
      n356 = Power Of X(1:w679, 2:0.2) -> (0:w731:dbl)
      n357 = Power Of X(1:w739, 2:0.2) -> (0:w792:dbl)
      n358 = Power Of X(1:2.718281828459045, 2:w554) -> (0:w552:dbl)
      n359 = Divide(x=w648, y=w656) -> (x/y=w640:dbl)
      n360 = Divide(x=w587, y=w595) -> (x/y=w579:dbl)
      n361 = Divide(x=w723, y=w731) -> (x/y=w715:dbl)
      n362 = Divide(x=w784, y=w792) -> (x/y=w776:dbl)
      n363 = Power Of X(1:2.718281828459045, 2:w690) -> (0:w688:dbl)
      n364 = Power Of X(1:2.718281828459045, 2:w751) -> (0:w749:dbl)
      n365 = Square(x=w640) -> (x^2=w634:dbl)
      n366 = Square(x=w579) -> (x^2=w573:dbl)
      n367 = Square(x=w715) -> (x^2=w709:dbl)
      n368 = Square(x=w776) -> (x^2=w770:dbl)
      n369 = Power Of X(1:w640, 2:3) -> (0:w633:dbl)
      n370 = Power Of X(1:w579, 2:3) -> (0:w572:dbl)
      n371 = Power Of X(1:w715, 2:3) -> (0:w708:dbl)
      n372 = Power Of X(1:w776, 2:3) -> (0:w769:dbl)
      n373 = Multiply(x=1.36603, y=w640) -> (x*y=w655:dbl)
      n374 = Multiply(x=1.36603, y=w579) -> (x*y=w594:dbl)
      n375 = Multiply(x=1.36603, y=w715) -> (x*y=w730:dbl)
      n376 = Multiply(x=1.36603, y=w776) -> (x*y=w791:dbl)
      n377 = Multiply(x=w633, y=0.11116) -> (x*y=w632:dbl)
      n378 = Multiply(x=w634, y=-0.47719) -> (x*y=w631:dbl)
      n379 = Multiply(x=w572, y=0.11116) -> (x*y=w571:dbl)
      n380 = Multiply(x=w573, y=-0.47719) -> (x*y=w570:dbl)
      n381 = Multiply(x=w708, y=0.11116) -> (x*y=w707:dbl)
      n382 = Multiply(x=w709, y=-0.47719) -> (x*y=w706:dbl)
      n383 = Multiply(x=w769, y=0.11116) -> (x*y=w768:dbl)
      n384 = Multiply(x=w770, y=-0.47719) -> (x*y=w767:dbl)
      n385 = Compound Arithmetic op=unknown(w632, w631, w655) -> (w607:dbl)
      n386 = Compound Arithmetic op=unknown(w571, w570, w594) -> (w547:dbl)
      n387 = Compound Arithmetic op=unknown(w707, w706, w730) -> (w683:dbl)
      n388 = Compound Arithmetic op=unknown(w768, w767, w791) -> (w743:dbl)
      n389 = Subtract(x=w601, y=w607) -> (x-y=w604:dbl)
      n390 = Multiply(x=w607, y=w609) -> (x*y=w608:dbl)
      n391 = Subtract(x=w541, y=w547) -> (x-y=w544:dbl)
      n392 = Multiply(x=w547, y=w536) -> (x*y=w548:dbl)
      n393 = Subtract(x=w677, y=w683) -> (x-y=w680:dbl)
      n394 = Multiply(x=w683, y=w672) -> (x*y=w684:dbl)
      n395 = Subtract(x=w737, y=w743) -> (x-y=w740:dbl)
      n396 = Multiply(x=w743, y=w745) -> (x*y=w744:dbl)
      n397 = Multiply(x=w613, y=w604) -> (x*y=w605:dbl)
      n398 = Multiply(x=w552, y=w544) -> (x*y=w545:dbl)
      n399 = Multiply(x=w688, y=w680) -> (x*y=w681:dbl)
      n400 = Multiply(x=w749, y=w740) -> (x*y=w741:dbl)
      n401 = Add(x=w605, y=w608) -> (x+y=w600:dbl)
      n402 = Add(x=w545, y=w548) -> (x+y=w540:dbl)
      n403 = Add(x=w681, y=w684) -> (x+y=w676:dbl)
      n404 = Add(x=w741, y=w744) -> (x+y=w736:dbl)
      n405 = Multiply(x=w600, y=w520) -> (x*y=w599:dbl)
      n406 = Multiply(x=w540, y=w520) -> (x*y=w539:dbl)
      n407 = Multiply(x=w676, y=w664) -> (x*y=w675:dbl)
      n408 = Multiply(x=w736, y=w664) -> (x*y=w735:dbl)
      n409 = Subtract(x=w601, y=w599) -> (x-y=w533:dbl)
      n410 = Subtract(x=w541, y=w539) -> (x-y=w532:dbl)
      n411 = Subtract(x=w677, y=w675) -> (x-y=w667:dbl)
      n412 = Subtract(x=w737, y=w735) -> (x-y=w668:dbl)
      n413 = case shown="False" w535 {
        tunnel: [w812 w818] -> w519
        tunnel: w520 -> [_ w819]
        tunnel: w534 -> [w815 _]
        tunnel: w533 -> [w814 _]
        tunnel: w532 -> [w813 _]
        frame False {
          n414 = case shown="False" w815 {
            tunnel: [w816 w817] -> w812
            tunnel: w814 -> [_ w817]
            tunnel: w813 -> [w816 _]
            frame False {
            }
            frame True {
            }
          }
        }
        frame True {
          n415 = Subtract(x=1.0, y=w819) -> (x-y=w818:dbl)
        }
      }
      n416 = case shown="False" w671 {
        tunnel: [w821 w827] -> w670
        tunnel: w664 -> [_ w828]
        tunnel: w669 -> [w824 _]
        tunnel: w668 -> [w823 _]
        tunnel: w667 -> [w822 _]
        frame False {
          n417 = case shown="False" w824 {
            tunnel: [w825 w826] -> w821
            tunnel: w823 -> [_ w826]
            tunnel: w822 -> [w825 _]
            frame False {
            }
            frame True {
            }
          }
        }
        frame True {
          n418 = Subtract(x=1.0, y=w828) -> (x-y=w827:dbl)
        }
      }
      n419 = Multiply(x=w519, y=w501) -> (x*y=w502:dbl)
      n420 = Multiply(x=w670, y=w512) -> (x*y=w511:dbl)
      n421 = case shown="False" w505 {
        tunnel: 0.0 -> [w797 w804]
        tunnel: w512 -> [w796 w811]
        tunnel: w511 -> [w795 w810]
        tunnel: "AFP Efficiency" -> [_ w798]
        tunnel: [w795 w806] -> w509
        tunnel: [w796 w805] -> w508
        tunnel: [w797 w804] -> w507
        tunnel: w502 -> [w794 w803]
        tunnel: [w794 w802] -> w503
        tunnel: w501 -> [w793 w801]
        tunnel: [w793 w799] -> w500
        frame False {
        }
        frame True {
          n422 = Negate(x=w801) -> (-x=w800:dbl)
          n423 = Negate(x=w803) -> (-x=w809:dbl)
          n424 = Negate(x=w810) -> (-x=w808:dbl)
          n425 = Negate(x=w811) -> (-x=w807:dbl)
          n426 = Multiply(x=w800, y=w798) -> (x*y=w799:dbl)
          n427 = Multiply(x=w809, y=w798) -> (x*y=w802:dbl)
          n428 = Multiply(x=w808, y=w798) -> (x*y=w806:dbl)
          n429 = Multiply(x=w807, y=w798) -> (x*y=w805:dbl)
        }
      }
    }
    n430 = Divide(x=12.0, y=500.0) -> (x/y=w103:dbl)
    n431 = Divide(x=12.0, y=500.0) -> (x/y=w141:dbl)
    n432 = Divide(x=12.0, y=500.0) -> (x/y=w145:dbl)
    n433 = Divide(x=12.0, y=500.0) -> (x/y=w99:dbl)
    n434 = Multiply(x=w95, y=w103) -> (x*y=→"upper R-value AFP":dbl)
    n435 = Multiply(x=w134, y=w141) -> (x*y=→"lower R-value":dbl)
    n436 = Multiply(x=w137, y=w145) -> (x*y=→"upper R-value":dbl)
    n437 = Multiply(x=w92, y=w99) -> (x*y=→"lower R-value AFP":dbl)
    n438 = case shown="True" w183 {
      tunnel: w187 -> [_ w489]
      tunnel: w86 -> [w485 w488]
      tunnel: w86 -> [_ w487]
      tunnel: [w485 w487] -> w186
      tunnel: [w484 w486] -> w174
      tunnel: w177 -> [w484 _]
      frame False {
      }
      frame True {
        n439 = Subtract(x=w489, y=w488) -> (x-y=w486:dbl[])
      }
    }
    n440 = case shown="True" w183 {
      tunnel: w201 -> [_ w495]
      tunnel: w192 -> [w491 w494]
      tunnel: w200 -> [_ w493]
      tunnel: [w491 w493] -> w184
      tunnel: [w490 w492] -> w173
      tunnel: w177 -> [w490 _]
      frame False {
      }
      frame True {
        n441 = Subtract(x=w495, y=w494) -> (x-y=w492:dbl[])
      }
    }
    n442 = Add(x=w186, y=w79) -> (x+y=w70:dbl[])
    n443 = Add(x=w174, y=w79) -> (x+y=w72:dbl[])
    n444 = Add(x=w80, y=w173) -> (x+y=w74:dbl[])
    n445 = Add(x=w80, y=w184) -> (x+y=w76:dbl[])
    n446 = call "FitAndSubtract.vi"("Array 4"=w67, "Array 3"=w68, "Numeric"=w69, "Array in"=w70) -> ("Array out"=w71:dbl[])  [unwired: 6 in, 1 out]
    n447 = call "FitAndSubtract.vi"("Array 4"=w67, "Array 3"=w68, "Numeric"=w69, "Array in"=w72) -> ("Array out"=w73:dbl[])  [unwired: 6 in, 1 out]
    n448 = call "FitAndSubtract.vi"("Array 4"=w67, "Array 3"=w68, "Numeric"=w69, "Array in"=w74) -> ("Array out"=w77:dbl[])  [unwired: 6 in, 1 out]
    n449 = Bundle(w68, w76) -> (w226:cluster{dbl[], dbl[]})  [unwired: 1 in]
    n450 = call "FitAndSubtract.vi"("Array 4"=w67, "Array 3"=w68, "Numeric"=w69, "Array in"=w76) -> ("Best Polynomial Fit"=w75:dbl[], "Array out"=w78:dbl[])  [unwired: 6 in]
    n451 = Bundle(w68, "Best Polynomial Fit"=w75) -> (w160:cluster{dbl[], "Best Polynomial Fit":dbl[]})  [unwired: 1 in]
    n452 = call "rhozero.vi"("Array in"=w71) -> ("Array out"=w181:dbl[])  [unwired: 10 in]
    n453 = call "rhominus.vi"("Array"=w78, "Array 2"=w71) -> ("Array 3"=w180:dbl[])  [unwired: 9 in]
    n454 = Add(x=w77, y=w73) -> (x+y=w175:dbl[])
    n455 = Subtract(x=w77, y=w73) -> (x-y=w176:dbl[])
    n456 = call "rhoplus.vi"("Array 3"=w71, "Array in"=w78) -> ("Array out"=w182:dbl[])  [unwired: 9 in]
    n457 = Build Array(w226, w160) -> (→"Signal and Fit (P)" →"Signal and Fit (P) 2":cluster{dbl[], "Best Polynomial Fit":dbl[]}[])
    n458 = Divide(x=w175, y=w172) -> (x/y=w171:dbl[])
    n459 = Subtract(x=w182, y=w181) -> (x-y=w169:dbl[])
    n460 = Divide(x=w176, y=w172) -> (x/y=w170:dbl[])
    n461 = Subtract(x=w181, y=w180) -> (x-y=w168:dbl[])
    n462 = Reverse 1D Array(array=w171) -> (reversed array=w179:dbl[])
    n463 = Reverse 1D Array(array=w170) -> (reversed array=w178:dbl[])
    n464 = Divide(x=w179, y=w172) -> (x/y=w83:dbl[])
    n465 = Divide(x=w178, y=w172) -> (x/y=w84:dbl[])
    n466 = Add(x=w168, y=w83) -> (x+y=w166:dbl[])
    n467 = Add(x=w169, y=w84) -> (x+y=w167:dbl[])
    n468 = Subtract(x=w167, y=w166) -> (x-y=w154:dbl[])
    n469 = Add(x=w166, y=w167) -> (x+y=w62:dbl[])
    n470 = Bundle(w68, w167) -> (w161:cluster{dbl[], dbl[]})  [unwired: 1 in]
    n471 = Bundle(w68, w166) -> (w162:cluster{dbl[], dbl[]})  [unwired: 1 in]
    n472 = Add Array Elements(numeric array=w62) -> (sum=w156:dbl)
    n473 = Add Array Elements(numeric array=w154) -> (sum=w155:dbl)
    n474 = Bundle(w68, w154) -> (→"Corrected Data (Q)":cluster{dbl[], dbl[]})  [unwired: 1 in]
    n475 = Bundle(w68, w62) -> (w163:cluster{dbl[], dbl[]})  [unwired: 1 in]
    n476 = Array To Spreadsheet String(delimiter (Tab)=",", array=w62, 3:"%f") -> (spreadsheet string=w66:string)
    n477 = Format Into String(format string="%d", initial string="", w56) -> (resulting string=w116:string)  [unwired: 1 in, 1 out]
    n478 = Build Array(w163, w161, w162) -> (→"Corrected Data (P)":cluster{dbl[], dbl[]}[])
    n479 = Number To Fractional String(number="Saturation\nPolarization", precision (6)=i16 2) -> (F-format string=w64:string)  [unwired: 2 in]
    n480 = Divide(x=12.0, y=500.0) -> (x/y=w152:dbl)
    n481 = Divide(x=12.0, y=500.0) -> (x/y=w146:dbl)
    n482 = Multiply(x=w156, y=w152) -> (x*y=w153:dbl)
    n483 = Multiply(x=w155, y=w146) -> (x*y=w149:dbl)
    n484 = Absolute Value(x=w153) -> (abs(x)=w106:dbl)
    "Reimann\nsum of P" <- w106
    n485 = Concatenate Strings(w116, ",", w64, ",", w66) -> (w113:string)
    n486 = Absolute Value(x=w149) -> (abs(x)=w133:dbl)
    "Reimann \nsum of Q" <- w133
    n487 = Write to Text File(file (use dialog)=w122, text=w113, error in=w121) -> (refnum out=w120:refnum<file>, error out=w119:errorcluster)  [unwired: 1 in, 1 out]
    n488 = Square(x=w106) -> (x^2=w104:dbl)
    n489 = Bundle(w106, w133) -> (→"Total Polarization (P)":cluster{dbl, dbl})  [unwired: 1 in]
    n490 = Quotient & Remainder(x=w56, y="Batch Size") -> (x-y*floor(x/y)=w54:i32)  [unwired: 1 out]
    n491 = Multiply(x=3, y=w104) -> (x*y=w108:dbl)
    n492 = Equal To 0?(x=w54) -> (x = 0?=w53:bool)
    n493 = Select(t="Training?", s=w53, f=FALSE) -> (s? t:f=w50:bool)
    n494 = call "Ann_int.vi"("Data"=w62, "Loss Function"="Loss Function", "Regularization"="Regularization", "Target"="Saturation\nPolarization", "Training?"=w50, "Parameters"=w60, "Adam Data In"=w57) -> ("Output"=w40:dbl, "Error"=w39:dbl, "Adjusted Parameters"=w46:T4, "Adam Data Out"=w58:T2)  [unwired: 4 in, 1 out]
    "NN Output" <- w40
    "NN Error" <- w39
    "NN Loss" <- w39
    "NN Output" <- w40
    "NN Error" <- w39
    n495 = Subtract(x=4, y=w108) -> (x-y=w105:dbl)
    n496 = call "Signal Production.vi"("Polarization"=w40) -> ("output cluster"=→"NN Graph":cluster{dbl[], "result":dbl[]})  [unwired: 10 in]
    n497 = Square Root(x=w105) -> (sqrt(x)=w110:dbl)
    n498 = Less?(x=w48, y=w39) -> (x < y?=w47:bool)
    n499 = Subtract(x=2, y=w110) -> ()  [unwired: 1 out]
    n500 = Select(t=w48, s=w47, f=w39) -> (s? t:f=w49:dbl)
    n501 = Select(t=w44, s=w47, f=w46) -> (s? t:f=w45:T4)
    "Saturation\nPolarization" <- "Saturation\nPolarization"
  }
  n502 = invoke class="VI" method="Default Vals.Reinit All"(reference=w38) -> ()  [unwired: 2 in, 3 out]
  n503 = property on="Total Polarization (P)" class="WFChart (strict)"("History Data"=cluster{dbl, dbl}[] []) -> ()  [unwired: 2 in, 2 out]
  n504 = property on="NN Training Loss" class="WFChart (strict)"("History Data"=dbl[] []) -> ()  [unwired: 2 in, 2 out]
  n505 = Close File(refnum=w34, error in=w33) -> ()  [unwired: 2 out]
  n506 = Flatten To XML(anything=w2) -> (xml string=w30:string)
  n507 = call-poly <vilib>:"Write to XML File.vi"("XML Input"=w30, "XML File Path"="Parameters File Path") -> ()  [unwired: 7 in, 3 out]
